vi "Servo LED Controlled By Encoder Accelerometer for Vibrations.vi"(8 "error in":errorcluster caption="Error In") -> (0 "Error Out":errorcluster)   [LabVIEW 2014]
doc: "Tested on:\n - Arduino Nano\n\nRotating servo motor there and back from 0deg to 180deg."
uses:
  LabVIEW-Universal-Transcriptor-ServoLibrary/ServoDatatype.lvclass
  <vilib>/LabVIEW Universal Transcriptor/LabVIEW to Arduino Transcriptor/Transcriptors/System API/Serial println string.vi
  <vilib>/LabVIEW Universal Transcriptor/Arduino MPU6050 Library/Arduino MPU6050.lvlib
  <vilib>/LabVIEW Universal Transcriptor/LabVIEW for Arduino Math Library/Arduino Math.lvlib
  <vilib>/LabVIEW Universal Transcriptor/LabVIEW Universal Transcriptor Rotary Encoder Library/Encoder.lvclass
panel:
  in  "encoder pin2":i32=7
  in  "encoder pin1":i32=6
  in  "address":u16(ring)=104 items=["AD0 pin NOT CONNECTED"=104, "AD0 connect to Vcc"=105]
  in  "range":T1(ring)
  in  "scale":T2(ring)
  in  "Servo Pin number":i32=4
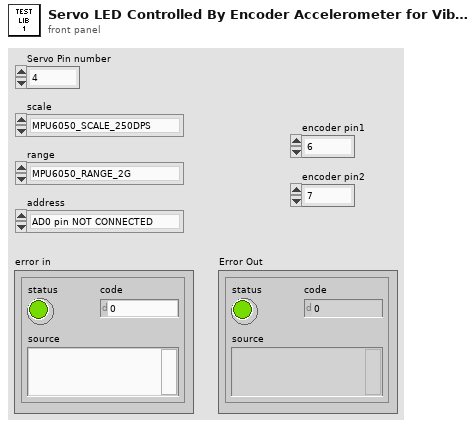
[diagram p1: front panel]
types:
  T1 = enum16{"MPU6050_RANGE_2G", "MPU6050_RANGE_4G", "MPU6050_RANGE_8G", "MPU6050_RANGE_16G"}
  T2 = enum16{"MPU6050_SCALE_250DPS", "MPU6050_SCALE_500DPS", "MPU6050_SCALE_1000DPS", "MPU6050_SCALE_2000DPS"}
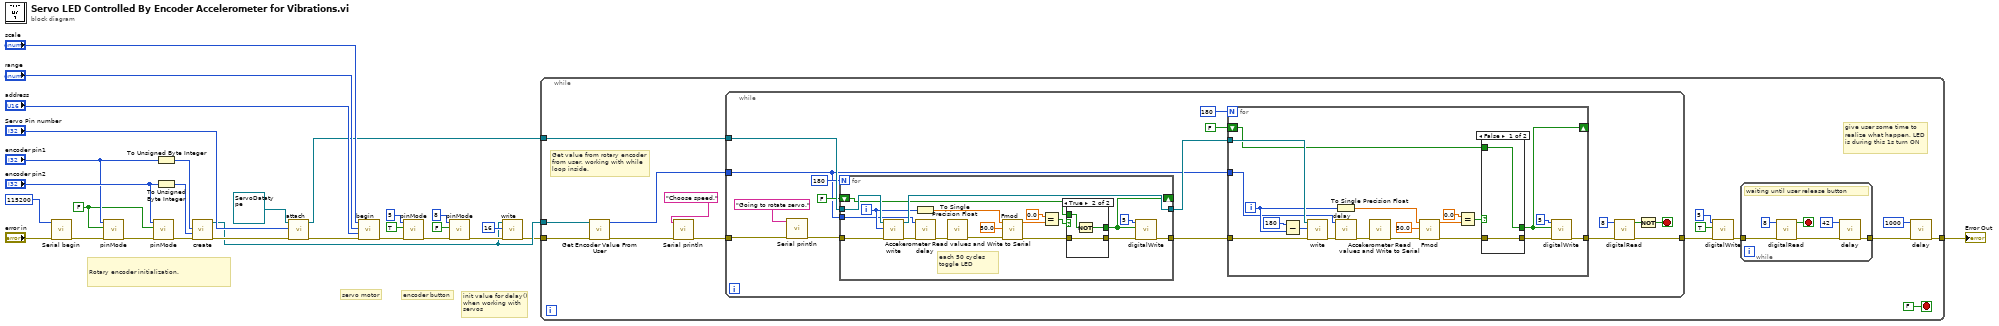
[diagram p0: block diagram]
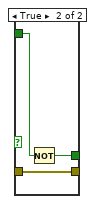
[diagram p2: hidden frame]
diagram:
  w12 = FALSE ("output?")
  # "servo motor"
  # "encoder button"
  # "init value for delay()\nwhen working with\nservos"
  # "Rotary encoder initialization."
  n1 = call <vilib>:"Serial begin.vi"("Error In"="error in", "speed (Bd)"=115200) -> ("Error Out"=w9:errorcluster)  [unwired: 9 in]
  n2 = call <vilib>:"pinMode.vi"("Error In"=w9, "output?"=w12, "pin number"="encoder pin1") -> ("Error Out"=w11:errorcluster)  [unwired: 8 in]
  n3 = call <vilib>:"pinMode.vi"("Error In"=w11, "output?"=w12, "pin number"="encoder pin2") -> ("Error Out"=w13:errorcluster)  [unwired: 8 in]
  n4 = To Unsigned Byte Integer(number="encoder pin1") -> (unsigned 8bit integer=w16:u8)
  n5 = To Unsigned Byte Integer(number="encoder pin2") -> (unsigned 8bit integer=w17:u8)
  n6 = call <vilib>:"create.vi"("error in"=w13, "pin2"=w17, "pin1"=w16) -> ("error out"=w18:errorcluster, "Encoder in"=w2:refnum<class "Encoder.lvclass">)  [unwired: 7 in]
  n7 = call-dynamic "attach.vi"("error in (no error)"=w18, "pin number"="Servo Pin number", "Servo in"=refnum<class "ServoDatatype.lvclass"> refnum) -> ("error out"=w24:errorcluster, "Servo out"=w23:refnum<class "ServoDatatype.lvclass">)  [unwired: 6 in, 1 out]
  n8 = call <vilib>:"begin.vi"("Error In"=w24, "address"="address", "range"="range", "scale"="scale") -> ("Error Out"=w21:errorcluster)  [unwired: 7 in]
  n9 = call <vilib>:"pinMode.vi"("Error In"=w21, "output?"=TRUE, "pin number"=5) -> ("Error Out"=w7:errorcluster)  [unwired: 8 in]
  n10 = call <vilib>:"pinMode.vi"("Error In"=w7, "output?"=FALSE, "pin number"=8) -> ("Error Out"=w4:errorcluster)  [unwired: 8 in]
  n11 = call <vilib>:"write.vi"("error in (no error)"=w4, "value"=16, "Encoder in"=w2) -> ("error out"=w1:errorcluster)  [unwired: 7 in]
  n12 = while {
    tunnel: w23 -> [w44]
    tunnel: w2 -> [w42]
    tunnel: w1 -> [w38]
    tunnel: [w43] -> w22
    stop <- FALSE stop-if-true
    # "give user some time to realize what happen, LED is during this 1s turn ON"
    # "Get value from rotary encoder\nfrom user, working with while\nloop inside."
    n13 = call "Get Encoder Value From User.vi"("error in (no error)"=w38, "Encoder in"=w42) -> ("error out"=w39:errorcluster, "Numeric"=w41:i32)  [unwired: 8 in]
    n14 = call-poly <vilib>:"Serial println.vi"("Error In"=w39, "string in"="Choose speed.") -> ("Error Out"=w40:errorcluster)  [unwired: 9 in]
    n15 = while {
      tunnel: w40 -> [w52]
      tunnel: w44 -> [w66]
      tunnel: [w55] -> w36
      tunnel: w41 -> [w59]
      stop <- w54 stop-if-true
      n16 = call-poly <vilib>:"Serial println.vi"("Error In"=w52, "string in"="Going to rotate servo.") -> ("Error Out"=w53:errorcluster)  [unwired: 9 in]
      n17 = for {
        N: 180 -> [_]
        tunnel: w66 -> [w110]
        tunnel: w53 -> [w95]
        tunnel: [w109] -> w65
        tunnel: [w100] -> w60
        shift-right: [w98] -> _
        shift-left: FALSE -> [w102]
        tunnel: w59 -> [w94]
        i -> [w108]
        # "each 50 cycles toggle LED"
        n18 = call-dynamic <vilib>:"write.vi"("error in (no error)"=w95, "value"=w108, "ServoDatatype in"=w110) -> ("error out"=w96:errorcluster, "ServoDatatype out"=w109:refnum<class "ServoDatatype.lvclass">)  [unwired: 7 in]
        n19 = To Single Precision Float(number=w108) -> (single precision float=w107:sgl)
        n20 = call <vilib>:"delay.vi"("Error In"=w96, "time (ms)"=w94) -> ("Error Out"=w93:errorcluster)  [unwired: 9 in]
        n21 = call "Accekerometer Read values and Write to Serial.vi"("error in (no error)"=w93) -> ("error out"=w92:errorcluster)  [unwired: 10 in]
        n22 = call <vilib>:"Fmod.vi"("Error In"=w92, "y"=sgl 50.0, "x"=w107) -> ("Error Out"=w106:errorcluster, "fmod(x,y)"=w104:sgl)  [unwired: 7 in]
        n23 = Equal?(x=sgl 0.0, y=w104) -> (x = y?=w105:bool)
        n24 = case shown="True" w105 {
          tunnel: w106 -> [w112 w113]
          tunnel: w102 -> [w111 w115]
          tunnel: [w112 w113] -> w99
          tunnel: [w111 w114] -> w98
          frame False {
          }
          frame True {
            n25 = Not(x=w115) -> (.not. x?=w114:bool)
          }
        }
        n26 = call <vilib>:"digitalWrite.vi"("Error In"=w99, "value"=w98, "pin number"=5) -> ("Error Out"=w100:errorcluster)  [unwired: 8 in]
      }
      n27 = for {
        N: 180 -> [_]
        tunnel: w65 -> [w86]
        tunnel: [w79] -> w56
        tunnel: w60 -> [w71]
        shift-right: [w77] -> _
        shift-left: FALSE -> [w81]
        tunnel: w59 -> [w69]
        i -> [w75]
        n28 = Subtract(x=180, y=w75) -> (x-y=w76:i32)
        n29 = call-dynamic <vilib>:"write.vi"("error in (no error)"=w71, "value"=w76, "ServoDatatype in"=w86) -> ("error out"=w70:errorcluster)  [unwired: 7 in, 1 out]
        n30 = To Single Precision Float(number=w75) -> (single precision float=w74:sgl)
        n31 = call <vilib>:"delay.vi"("Error In"=w70, "time (ms)"=w69) -> ("Error Out"=w68:errorcluster)  [unwired: 9 in]
        n32 = call "Accekerometer Read values and Write to Serial.vi"("error in (no error)"=w68) -> ("error out"=w67:errorcluster)  [unwired: 10 in]
        n33 = call <vilib>:"Fmod.vi"("Error In"=w67, "y"=sgl 50.0, "x"=w74) -> ("Error Out"=w82:errorcluster, "fmod(x,y)"=w83:sgl)  [unwired: 7 in]
        n34 = Equal?(x=sgl 0.0, y=w83) -> (x = y?=w73:bool)
        n35 = case shown="False" w73 {
          tunnel: [w88 w89] -> w80
          tunnel: w82 -> [w88 w89]
          tunnel: w81 -> [w87 w91]
          tunnel: [w87 w90] -> w77
          frame False {
          }
          frame True {
            n36 = Not(x=w91) -> (.not. x?=w90:bool)
          }
        }
        n37 = call <vilib>:"digitalWrite.vi"("Error In"=w80, "value"=w77, "pin number"=5) -> ("Error Out"=w79:errorcluster)  [unwired: 8 in]
      }
      n38 = call <vilib>:"digitalRead.vi"("Error In"=w56, "pin number"=8) -> ("Error Out"=w55:errorcluster, "value"=w57:bool)  [unwired: 8 in]
      n39 = Not(x=w57) -> (.not. x?=w54:bool)
    }
    n40 = call <vilib>:"digitalWrite.vi"("Error In"=w36, "value"=TRUE, "pin number"=5) -> ("Error Out"=w34:errorcluster)  [unwired: 8 in]
    n41 = while {
      tunnel: w34 -> [w48]
      tunnel: [w46] -> w33
      stop <- w49 stop-if-true
      # "waiting until user release button"
      n42 = call <vilib>:"digitalRead.vi"("Error In"=w48, "pin number"=8) -> ("Error Out"=w47:errorcluster, "value"=w49:bool)  [unwired: 8 in]
      n43 = call <vilib>:"delay.vi"("Error In"=w47, "time (ms)"=42) -> ("Error Out"=w46:errorcluster)  [unwired: 9 in]
    }
    n44 = call <vilib>:"delay.vi"("Error In"=w33, "time (ms)"=1000) -> ("Error Out"=w43:errorcluster)  [unwired: 9 in]
  }
  "Error Out" <- w22
